vi "Main.vi"(11 "Module Admin":refnum<class "Delacor_lib_QMH_Module Admin.lvclass">) -> ()   [LabVIEW 2019, in "SME_Data_Acquisition.lvlib"]
doc: "This template is based off of the Queued Message Handler design pattern and the Queued Message Handler project template that ships with LabVIEW.\n\nThe main difference is that the queue is private to this module and communication between modules is performed via Broadcast and Request events.\n\nRequest events are wrapped in public API methods and are handled in the Event Handling Loop (EHL) of this VI. Any module can register for Broadcast events sent by this module. The EHL generates messages based on user interface actions.\n\nThe Message Handling Loop (MHL) processes messages generated by the EHL, or by other messages. The messages are string values, so new messages can be added easily to the Message Cases case structure in the MHL. Each message cluster can also provide an optional value for Message Data, which is a variant that can be converted to whatever message-specific data is required.\n_____\nBased on DQMH Project Template 7.0.1.1316."
uses:
  SME_Data_Acquisition.lvlib
  <vilib>/Delacor/Delacor QMH/Libraries/Module Admin_class/Delacor_lib_QMH_Module Admin.lvclass
  Module Data--cluster.ctl
  <vilib>/Delacor/Delacor QMH/Libraries/Message Queue_class/Delacor_lib_QMH_Message Queue.lvclass/Delacor_lib_QMH_Message Queue.ctl
  Stop Argument--cluster.ctl
  <vilib>/Delacor/Delacor QMH/Libraries/Module Admin_class/Delacor_lib_QMH_Module Admin.lvclass/Delacor_lib_QMH_Module Admin.ctl
  LogData Argument--cluster.ctl
  04 Class/Protocol/Protocol.lvclass
  <vilib>/Utility/sysdir.llb/System Directory Type.ctl
  <vilib>/Delacor/Delacor QMH/Libraries/Message Queue_class/Delacor_lib_QMH_Enqueue Message (Single).vi
  <vilib>/Delacor/Delacor QMH/Libraries/Module Admin_class/Delacor_lib_QMH_Get External Launch.vi
  <vilib>/Utility/file.llb/Write Delimited Spreadsheet (string).vi
  <vilib>/Delacor/Delacor QMH/Libraries/Message Queue_class/Delacor_lib_QMH_Message Queue.lvclass
panel:
  in  "Close":bool
  in  "LogEnable":bool caption="Data Log"
  in  "Com_Set":T1
  out "StatusLED":bool
  in  "Connect":bool
  in  "Protocol":enum16{"RS-232", "TCP/IP", "Modbus TCP/IP"}(ring)
  in  "Path":path caption="File Path"
  out "Data_Cluster":T2 {"Coil Temperature" format="%.2f"; "Channel 2 (c2)" format="%.3f"; "Channel 1 (c1)" format="%.3f"; "Freqency +45 Deg" format="%.7f"; "Freqency -45 Deg" format="%.7f"; "Freqency 0 Deg" format="%.7f"; "df frequency quotient" format="%.7f"; "Density" format="%.3f"; "Viscosity" format="%.3f"; "Damping Frequency" format="%.2g"; "Resonant Frequency" format="%.2f"; "Temperature" format="%.2f"}
  out "Table":string[][](table)
  out "Chart1":cluster{"Viscosity":dbl, "Temperature":dbl}(graph)
  out "Chart2":cluster{"Viscosity":dbl, "Temperature":dbl}(graph)
  out "Chart3":cluster{"Viscosity":dbl, "Temperature":dbl}(graph)
  out "ReceivedData":string
  out "error out":errorcluster
  out "Status":string
  in  "Simulate MHL Error":bool
  in  "Simulate EHL Error":bool
  # "Data Acquisition Interface"
  # "Other processes communicate with this Module via its Public API (wrappers for its Request Events).\n\nThis Module communicates with other processes via its Broadcast Events.\nAny process that wants to receive these messages can register for this module's Broadcast events."
  # "This template is for the DQMH framework. See the block diagram for more information on how to use this template."
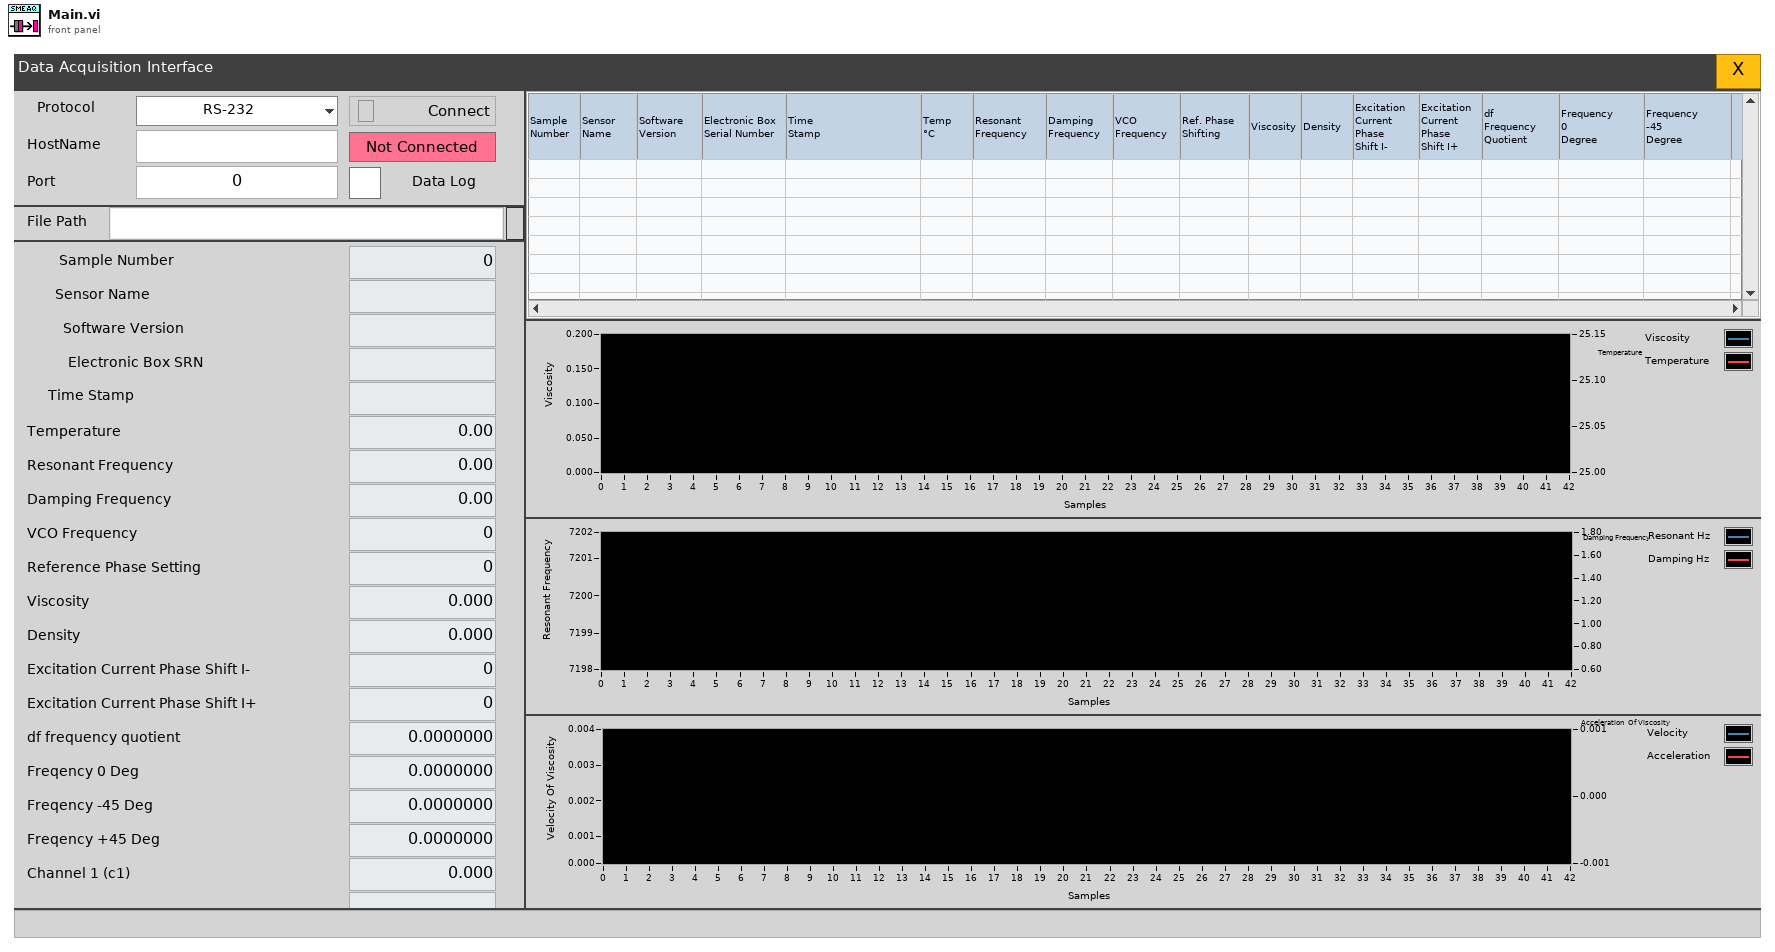
[diagram p1: front panel]
types:
  T1 = cluster{"HostName":string, "Port":dbl, "ComPort":string}
  T2 = cluster{"Sample Number":u16, "Sensor Name":string, "Software Version":string, "Electronic Box SRN":string, "Time Stamp":string, "Temperature":dbl, "Resonant Frequency":dbl, "Damping Frequency":dbl, "VCO Frequency":u16, "Reference Phase Setting":u16, "Viscosity":dbl, "Density":dbl, "Excitation Current Phase Shift I-":u16, "Excitation Current Phase Shift I+":u16, "df frequency quotient":dbl, "Freqency 0 Deg":dbl, "Freqency -45 Deg":dbl, "Freqency +45 Deg":dbl, "Channel 1 (c1)":dbl, "Channel 2 (c2)":dbl, "Coil Temperature":dbl, "Error State":u8}
  T3 = typedef "SME_Data_Acquisition.lvlib/Request Events--cluster.ctl" = cluster{"Stop Module":refnum<user-event>, "Show Panel":refnum<user-event>, "Hide Panel":refnum<user-event>, "Get Module Execution Status":refnum<user-event>, "Show Diagram":refnum<user-event>, "Private":cluster{"LogData":refnum<user-event>}}
  T4 = typedef "SME_Data_Acquisition.lvlib/Module Data--cluster.ctl" = cluster{"Status":string, "Path":refnum<vi>}
  T5 = cluster{"HostName":string, "Port":u16, "ComPort":string}
  T6 = enum32{"invalid lock state", "Not Locked", "Locked (No Password)", "Password-protected"}
  T7 = typedef "SME_Data_Acquisition.lvlib/Stop Argument--cluster.ctl" = cluster{"Origin":string, "Exit via Stop Module Req?":bool, "Wait for Module to stop?":bool}
  T8 = typedef "SME_Data_Acquisition.lvlib/LogData Argument--cluster.ctl" = cluster{"Data_Cluster":cluster{"Sample Number":u16, "Sensor Name":string, "Software Version":string, "Electronic Box SRN":string, "Time Stamp":string, "Temperature":dbl, "Resonant Frequency":dbl, "Damping Frequency":dbl, "VCO Frequency":u16, "Reference Phase Setting":u16, "Viscosity":dbl, "Density":dbl, "Excitation Current Phase Shift I-":u16, "Excitation Current Phase Shift I+":u16, "df frequency quotient":dbl, "Freqency 0 Deg":dbl, "Freqency -45 Deg":dbl, "Freqency +45 Deg":dbl, "Channel 1 (c1)":dbl, "Channel 2 (c2)":dbl, "Coil Temperature":dbl, "Error State":u8}}
  T9 = enum8{"Enabled", "Disabled", "Disabled and Grayed Out"}
  T10 = enum16{"Always On", "Always Off", "Off While Running"}
  T11 = enum32{"Invalid", "Standard", "Closed", "Hidden", "Minimized", "Maximized"}
  T12 = typedef "LVRectTypeDef.ctl" = cluster{"Left":i16, "Top":i16, "Right":i16, "Bottom":i16}
  T13 = typedef "System Directory Type.ctl" = i32
  T14 = cluster{"This VI":refnum<vi>, "ProtocolCls":refnum<class "Protocol.lvclass">, "Stream":string, "Table":refnum<vi>, "Data":string[][], "StatusLED":refnum<vi>, "LimitRowCount":u16, "Chart1":refnum<vi>, "Chart2":refnum<vi>, "Chart3":refnum<vi>, "Protocol":refnum<vi>, "Connect":refnum<vi>, "Com_Set":refnum<vi>, "Data_Cluster":refnum<vi>, "ConOpen":bool, "LogEnable":refnum<vi>}
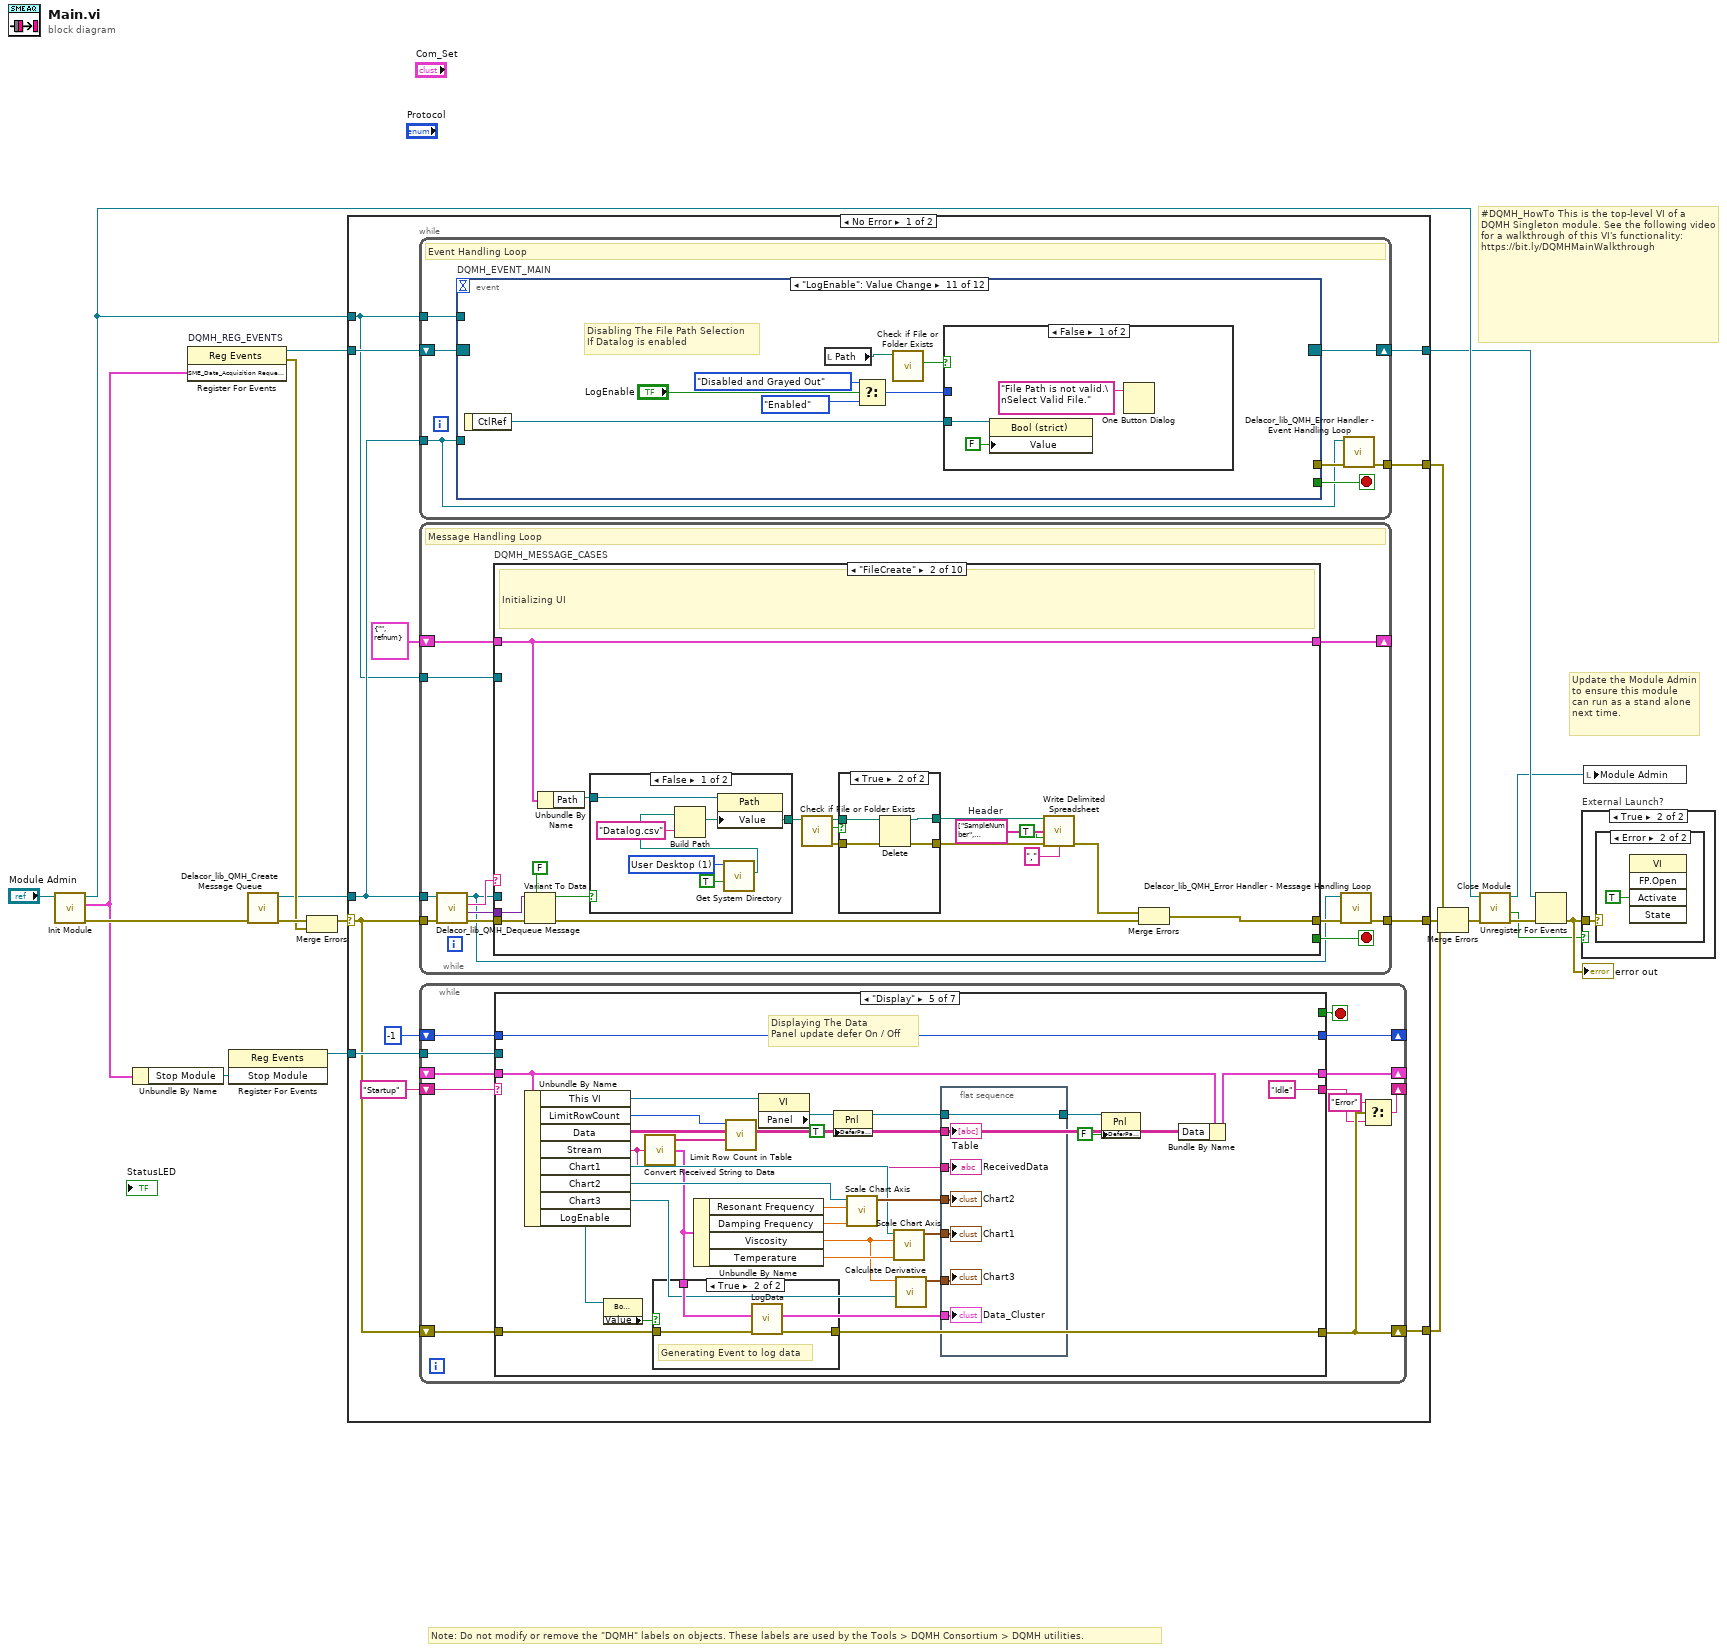
[diagram p0: block diagram]
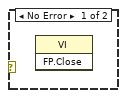
[diagram p3: hidden frame]
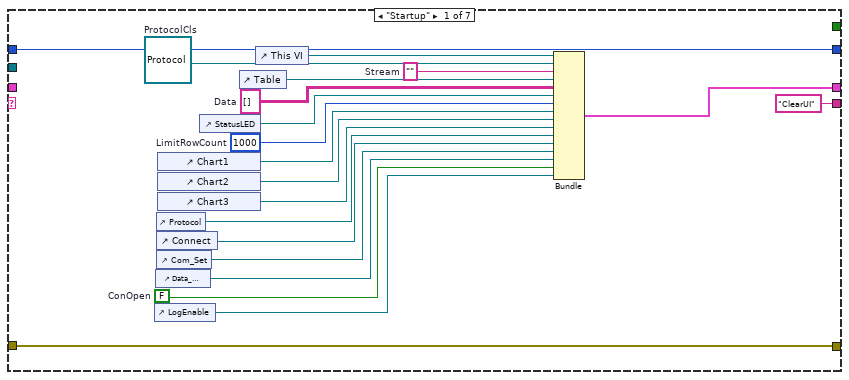
[diagram p4: hidden frame]
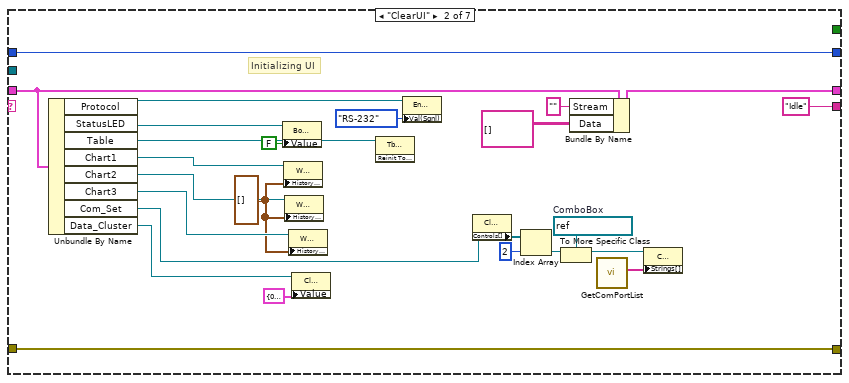
[diagram p5: hidden frame]
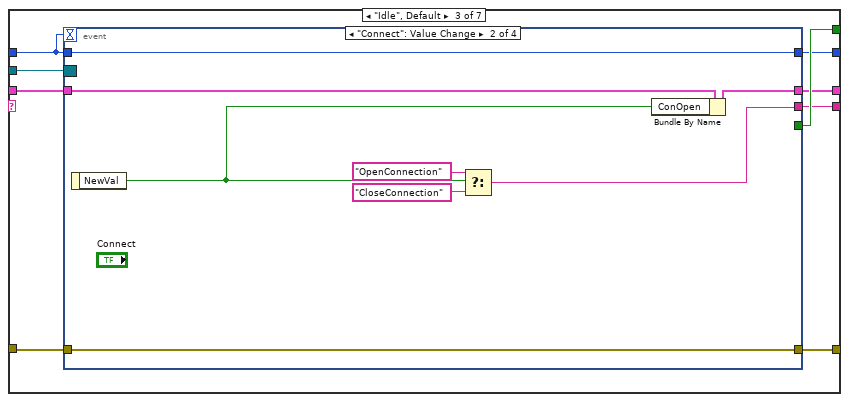
[diagram p6: hidden frame]
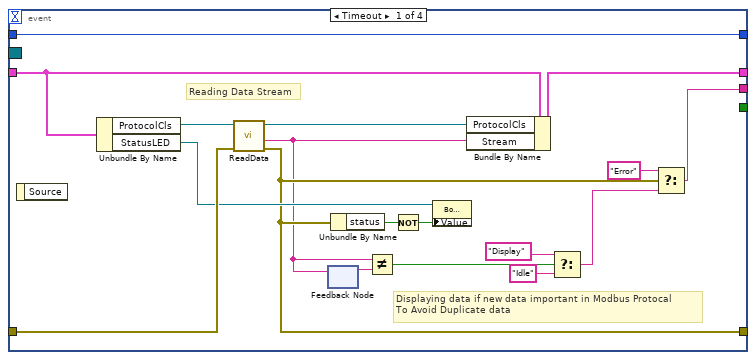
[diagram p7: hidden frame]
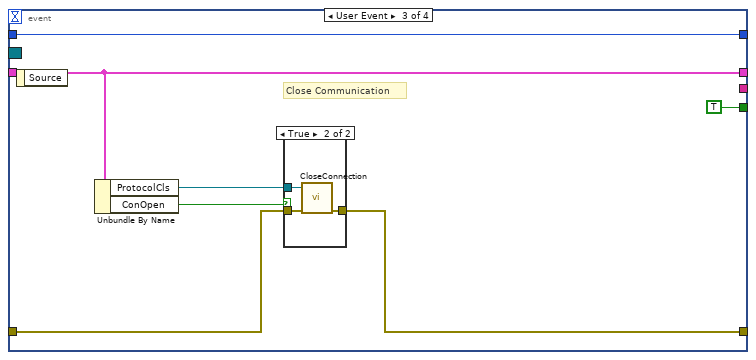
[diagram p8: hidden frame]
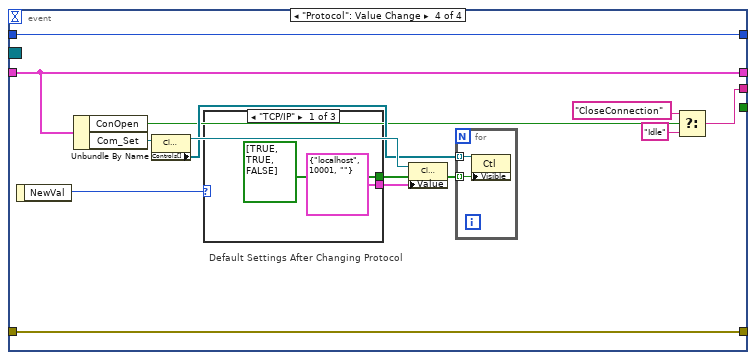
[diagram p10: hidden frame]
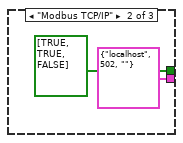
[diagram p11: hidden frame]
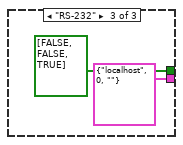
[diagram p12: hidden frame]
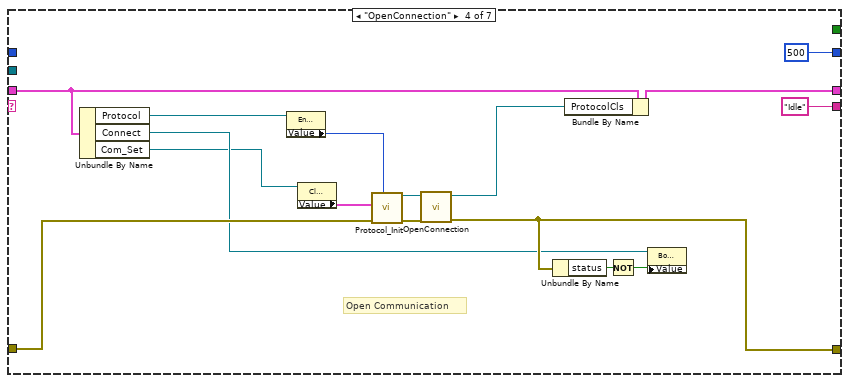
[diagram p13: hidden frame]
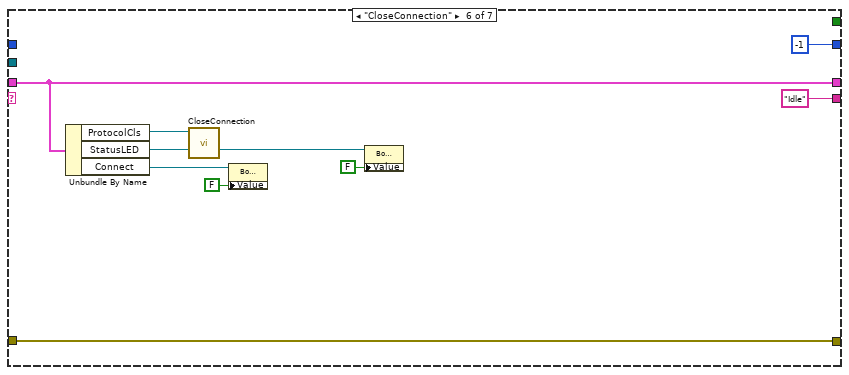
[diagram p15: hidden frame]
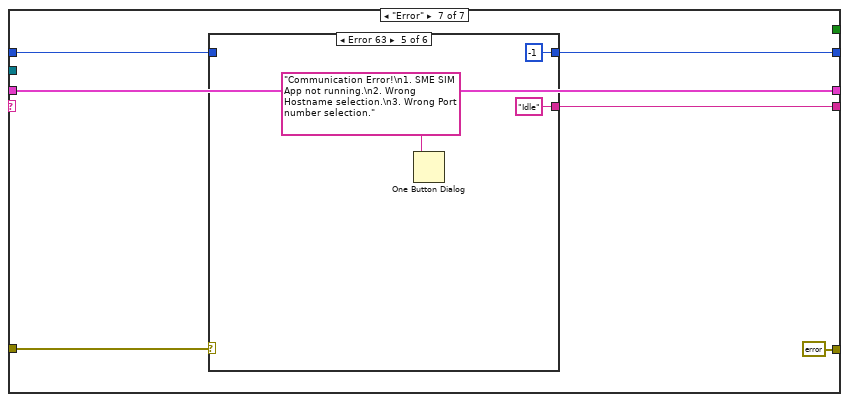
[diagram p16: hidden frame]
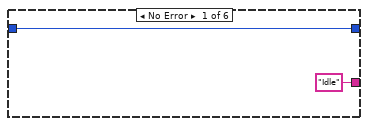
[diagram p17: hidden frame]
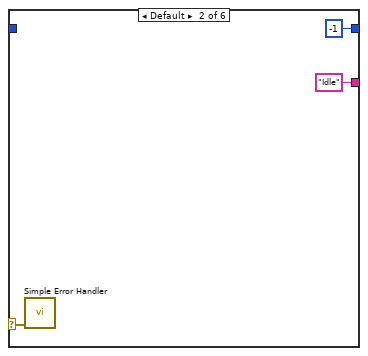
[diagram p18: hidden frame]
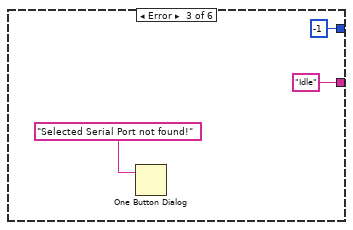
[diagram p19: hidden frame]
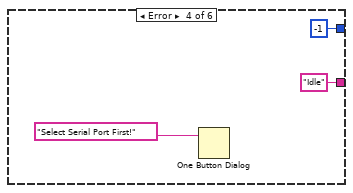
[diagram p20: hidden frame]
diagram:
  # "#DQMH_HowTo This is the top-level VI of a DQMH Singleton module. See the following video for a walkthrough of this VI's functionality: https://bit.ly/DQMHMainWalkthrough"
  # "Note: Do not modify or remove the \"DQMH\" labels on objects. These labels are used by the Tools > DQMH Consortium > DQMH utilities."
  # "Update the Module Admin to ensure this module can run as a stand alone next time."
  n1 = call "Init Module.vi"("Singleton Module Admin in"="Module Admin") -> ("error out"=w19:errorcluster, "SME_Data_Acquisition Request Events"=w4:T3, "Singleton Module Admin out"=w11:refnum<class "Delacor_lib_QMH_Module Admin.lvclass">)  [unwired: 8 in]
  n2 = Unbundle By Name(w4) -> ("Stop Module"=w3:refnum<user-event>)
  n3 = register-events "DQMH_REG_EVENTS"(w4) -> (reference out=w9:refnum<event-registration>, error out=w12:errorcluster)  [unwired: 2 in]
  n4 = register-events(w3) -> (reference out=w2:refnum<event-registration>)  [unwired: 2 in, 1 out]
  n5 = call <vilib>:"Delacor_lib_QMH_Create Message Queue.vi"("error in"=w19) -> ("error out"=w14:errorcluster, "Message Queue"=w8:refnum<class "Delacor_lib_QMH_Message Queue.lvclass">)  [unwired: 9 in]
  n6 = Merge Errors(w14, w12) -> (w13:errorcluster)
  n7 = case shown="No Error" w13 {
    selector: w13 -> [w22 w515]
    tunnel: [w32 w514] -> w20
    tunnel: [w30 w513] -> w10
    tunnel: w9 -> [w28 w513]
    tunnel: w8 -> [w27 w508]
    tunnel: [w31 _] -> w17
    tunnel: w11 -> [w26 w509]
    tunnel: w2 -> [w24 _]
    tunnel: [w21 _] -> w1
    frame No Error {
      n8 = while {
        tunnel: w27 -> [w245]
        shift-right: [w248] -> w30
        shift-left: w28 -> [w249]
        tunnel: [w250] -> w31
        tunnel: w26 -> [w246]
        stop <- w247 stop-if-true
        # "Event Handling Loop"
        n9 = event "DQMH_EVENT_MAIN" shown="[10] \"LogEnable\": Value Change" {
          selector: w249 -> [_ _ _ _ _ _ _ _ _ _ _ _]
          dyn-events: [_ _ _ _ _ _ _ _ _ _ _ _] -> w248
          timeout: _ -> [_ _ _ _ _ _ _ _ _ _ _ _]
          tunnel: [_ _ _ _ _ _ TRUE ("Discard?") _ _ _ _ _] -> w247
          tunnel: w245 -> [_ w259 _ _ _ _ w283 w290 w302 w316 _ w329]
          tunnel: [w257 w260 _ _ w266 _ w286 w292 w303 w311 _ _] -> w251
          tunnel: w246 -> [_ _ _ _ _ _ _ w289 w301 _ _ _]
          event "Simulate EHL Error": Value Change {
            # "#DQMH_HowTo The 'Simulate EHL Error' button  illustrates how the EHL handles errors. This event is instructional in nature and can be removed."
            # "This case simulates an error being generated by the EHL"
            n10 = event-data() -> ()  [unwired: 1 in, 1 out]
            n11 = call "Module Name--constant.vi"() -> ("Module Name"=w254:string)  [unwired: 11 in]
            n12 = Format Into String(format string="Simulated error originating at Event Handling Loop in %s", w254) -> (resulting string=w255:string)  [unwired: 2 in, 1 out]
            n13 = call <vilib>:"Error Cluster From Error Code.vi"("show call chain? (False)"=TRUE, "error message (\"\")"=w255, "error code (0)"=5000) -> ("error out"=w257:errorcluster)  [unwired: 6 in]
          }
          event "Simulate MHL Error": Value Change {
            # "#DQMH_HowTo The 'Simulate MHL Error' button  illustrates how the MHL handles errors. This event is instructional in nature and can be removed."
            # "This case simulates an error being generated by the MHL"
            n14 = event-data() -> ()  [unwired: 1 in, 1 out]
            n15 = call-poly <vilib>:"Delacor_lib_QMH_Enqueue Message (poly).vi"("Message"="Simulate MHL Error", "Message Queue in"=w259) -> ("error out"=w260:errorcluster)  [unwired: 8 in, 1 out]
          }
          event User Event {
            # "Show the panel of this VI, and send a status updated message to let listeners know."
            # "Another Module called the \"Show Panel\" API Method."
            n16 = event-data() -> ()  [unwired: 1 in, 1 out]
            n17 = control-ref of="This VI"() -> (w262:refnum<vi>)
            n18 = call "Open VI Panel.vi"("VI"=w262) -> ()  [unwired: 10 in, 1 out]
            n19 = call "Status Updated.vi"("Status"="Panel shown." ("format string")) -> ()  [unwired: 10 in, 1 out]
          }
          event User Event {
            # "Hide the panel of this VI, and send a status updated message to let listeners know."
            # "Another Module called the \"Hide Panel\" API Method."
            n20 = event-data() -> ()  [unwired: 1 in, 1 out]
            n21 = control-ref of="This VI"() -> (w264:refnum<vi>)
            n22 = call "Hide VI Panel.vi"("VI"=w264) -> ()  [unwired: 10 in, 1 out]
            n23 = call "Status Updated.vi"("Status"="Panel hidden." ("format string")) -> ()  [unwired: 10 in, 1 out]
          }
          event User Event {
            # "Another Module called the \"Get Module Execution Status\" API Method."
            n24 = event-data() -> ()  [unwired: 1 in, 1 out]
            n25 = call "Update Module Execution Status.vi"("Running?"=TRUE) -> ("error out"=w266:errorcluster)  [unwired: 10 in]
          }
          event User Event {
            # "Another Module called the \"Show Diagram\" API Method. This event is used for debugging."
            n26 = event-data() -> ()  [unwired: 1 in, 1 out]
            n27 = disable-structure shown="RUN_TIME_ENGINE==False" {
              frame condition #0 (active) {
                # "functionality not available in exe"
                n28 = invoke on="Invoke Node" class="VI" method="Lock State.Get"() -> (error out=w272:errorcluster, "Get Lock State"=w271:T6, "pwd in cache"=w268:bool)  [unwired: 4 in, 1 out]
                n29 = Equal?(x=T6."Password-protected", y=w271) -> (x = y?=w269:bool)
                n30 = Compound Arithmetic op=AND(w269, invert w268) -> (w267:bool)
                n31 = case shown="False" w267 {
                  tunnel: w272 -> [w275 _]
                  frame False {
                    n32 = property on="Property Node" class="VI"(error in=w275, "BDWin.Open"=TRUE ("Block Diagram Window:Open")) -> ()  [unwired: 1 in, 2 out]
                    n33 = call "Status Updated.vi"("Status"="Block Diagram shown." ("format string")) -> ()  [unwired: 10 in, 1 out]
                  }
                  frame True {
                    # "Password-protected VI, and the password is not in the cache. Do not show the diagram."
                  }
                }
              }
              frame condition #1 {
              }
            }
          }
          event User Event {
            # "The Stop Module Event can get fired from the Exit message in the MHL. The queue gets destroyed in that case. If the queue no longer exists, the Enqueue Exit as a priority message will return error 1. It is safe to ignore, because the module is already exiting."
            # "Another Module called the \"Stop Module\" API Method  or the Message Handling Loop below."
            n34 = event-data() -> ("Origin"=w282:string, "Exit via Stop Module Req?"=w278:bool, "Wait for Module to stop?"=w277:bool)  [unwired: 1 in]
            n35 = local write "Status"(w282) -> ()
            n36 = Bundle By Name(cluster=T7 {"Origin"="", "Exit via Stop Module Req?"=FALSE, "Wait for Module to stop?"=FALSE} ("Stop Argument"), "Exit via Stop Module Req?"=w278, "Wait for Module to stop?"=w277) -> (w276:T7)
            n37 = call-poly <vilib>:"Delacor_lib_QMH_Enqueue Message (poly).vi"("Priority Message? (F)"=TRUE, "Message Data"=w276, "Message"="Exit", "Message Queue in"=w283) -> ("error out"=w287:errorcluster)  [unwired: 6 in, 1 out]
            n38 = call <vilib>:"Clear Errors.vi"("error in (no error)"=w287, "specific error code to clear (0: all)"=1) -> ("error out"=w286:errorcluster)  [unwired: 4 in, 1 out]
          }
          event Panel Close? {
            w291 = TRUE  # Discard the event, the MHL is responsible for closing and stopping this VI.
            # "Hide the panel or send the 'Exit' message if the user clicks the 'X' on the module main VI panel."
            n39 = event-data() -> ()  [unwired: 1 in, 1 out]
            n40 = property on="Property Node" class="Module Admin"(reference=w289) -> ("Accessors:External Launch"=w288:bool)  [unwired: 1 in, 2 out]
            n41 = case shown="False" w288 {
              tunnel: w290 -> [_ w298]
              tunnel: [_ w299] -> w292
              frame True {
                # "If externally launched, clicking the 'X' hides the panel, but doesn't close it."
                n42 = control-ref of="This VI"() -> (w295:refnum<vi>)
                n43 = call "Hide VI Panel.vi"("VI"=w295) -> ("error out"=w293:errorcluster)  [unwired: 10 in]
                n44 = call "Status Updated.vi"("error in"=w293, "Status"="Panel hidden." ("format string")) -> ()  [unwired: 9 in, 1 out]
              }
              frame False {
                # "If run as a stand-alone VI, clicking the panel 'X' stops the VI."
                n45 = call-poly <vilib>:"Delacor_lib_QMH_Enqueue Message (poly).vi"("Priority Message? (F)"=TRUE, "Message"="Exit", "Message Queue in"=w298) -> ("error out"=w299:errorcluster)  [unwired: 7 in, 1 out]
              }
            }
            n46 = event-data ("Event Filter Node")("Discard?"=w291) -> ()  [unwired: 1 in, 1 out]
          }
          event "Close": Value Change {
            # "Hide the panel or send the 'Exit' message if the user clicks the 'X' on the module main VI panel."
            n47 = event-data() -> ()  [unwired: 1 in, 1 out]
            n48 = property on="Property Node" class="Module Admin"(reference=w301) -> ("Accessors:External Launch"=w300:bool)  [unwired: 1 in, 2 out]
            n49 = case shown="False" w300 {
              tunnel: w302 -> [_ w309]
              tunnel: [_ w310] -> w303
              frame True {
                # "If externally launched, clicking the 'X' hides the panel, but doesn't close it."
                n50 = control-ref of="This VI"() -> (w306:refnum<vi>)
                n51 = call "Hide VI Panel.vi"("VI"=w306) -> ("error out"=w304:errorcluster)  [unwired: 10 in]
                n52 = call "Status Updated.vi"("error in"=w304, "Status"="Panel hidden." ("format string")) -> ()  [unwired: 9 in, 1 out]
              }
              frame False {
                # "If run as a stand-alone VI, clicking the panel 'X' stops the VI."
                n53 = call-poly <vilib>:"Delacor_lib_QMH_Enqueue Message (poly).vi"("Priority Message? (F)"=TRUE, "Message"="Exit", "Message Queue in"=w309) -> ("error out"=w310:errorcluster)  [unwired: 7 in, 1 out]
              }
            }
          }
          event User Event {
            # "This module called the \"Private.LogData\" private request."
            n54 = event-data() -> ("Data_Cluster"=w312:T2)  [unwired: 1 in]
            n55 = Bundle(cluster=T8 {"Data_Cluster"={"Sample Number"=0, "Sensor Name"="", "Software Version"="", "Electronic Box SRN"="", "Time Stamp"="", "Temperature"=0.0, "Resonant Frequency"=0.0, "Damping Frequency"=0.0, "VCO Frequency"=0, "Reference Phase Setting"=0, "Viscosity"=0.0, "Density"=0.0, "Excitation Current Phase Shift I-"=0, "Excitation Current Phase Shift I+"=0, "df frequency quotient"=0.0, "Freqency 0 Deg"=0.0, "Freqency -45 Deg"=0.0, "Freqency +45 Deg"=0.0, "Channel 1 (c1)"=0.0, "Channel 2 (c2)"=0.0, "Coil Temperature"=0.0, "Error State"=0}} ("LogData Argument"), "Data_Cluster"=w312) -> (w313:T8)
            n56 = call-poly <vilib>:"Delacor_lib_QMH_Enqueue Message (poly).vi"("Message Data"=w313, "Message"="LogData", "Message Queue in"=w316) -> ("error out"=w311:errorcluster)  [unwired: 7 in, 1 out]
          }
          event "LogEnable": Value Change {
            # "Disabling The File Path Selection\nIf Datalog is enabled"
            n57 = event-data() -> ("CtlRef"=w317:refnum<vi>)  [unwired: 1 in]
            n58 = local read "Path"() -> (w319:path)
            n59 = Select(t=T9."Disabled and Grayed Out" ("Disabled"), s="LogEnable", f=T9."Enabled" ("Disabled")) -> (s? t:f=w320:T9)
            n60 = call <vilib>:"Check if File or Folder Exists.vi"("path"=w319) -> ("file or folder exists?"=w318:bool)  [unwired: 8 in, 2 out]
            n61 = case shown="False" w318 {
              tunnel: w320 -> [_ w327]
              tunnel: w317 -> [w325 _]
              frame False {
                n62 = property class="Bool (strict)"(reference=w325, "Value"=FALSE) -> ()  [unwired: 1 in, 2 out]
                n63 = One Button Dialog(message="File Path is not valid.\nSelect Valid File.") -> ()  [unwired: 1 in, 1 out]
              }
              frame True {
                n64 = property on="Path" class="Path"("DisabledEnum"=w327) -> ()  [unwired: 2 in, 2 out]
              }
            }
          }
          event "Path": Value Change {
            w328 = TRUE  # PathChangedByUser
            # "Sending"
            n65 = event-data() -> ()  [unwired: 1 in, 1 out]
            n66 = call-poly <vilib>:"Delacor_lib_QMH_Enqueue Message (poly).vi"("Message Data"=w328, "Message"="FileCreate", "Message Queue in"=w329) -> ()  [unwired: 7 in, 2 out]
          }
        }
        n67 = call-dynamic "Delacor_lib_QMH_Error Handler - Event Handling Loop.vi"("error in"=w251, "Message Queue in"=w245) -> ("dup error in"=w250:errorcluster)  [unwired: 8 in, 1 out]
      }
      n68 = while {
        tunnel: w27 -> [w331]
        shift-right: [w339] -> _
        shift-left: T4 {"Status"="", "Path"=refnum} ("Data Cluster") -> [w340]
        tunnel: w22 -> [w342]
        tunnel: [w334] -> w32
        tunnel: w26 -> [w335]
        stop <- w338 stop-if-true
        # "Message Handling Loop"
        n69 = call-dynamic "Delacor_lib_QMH_Dequeue Message.vi"("error in"=w342, "Message Queue in"=w331) -> ("error out"=w341:errorcluster, "Message Data"=w336:variant, "Message"=w337:string, "Message Queue out"=w332:refnum<class "Delacor_lib_QMH_Message Queue.lvclass">)  [unwired: 6 in]
        n70 = case "DQMH_MESSAGE_CASES" shown="\"FileCreate\"" w337 {
          selector: w337 -> [_ _ _ _ _ _ _ _ _ w503]
          tunnel: w332 -> [w359 _ _ _ _ _ _ w469 w491 _]
          tunnel: w341 -> [w375 w384 w410 w451 w454 w456 w465 w476 w497 w506]
          tunnel: [w358 w379 w410 w412 w453 w456 w464 w472 w492 w507] -> w333
          tunnel: w340 -> [w367 w394 w409 w446 w452 w455 w462 w471 w490 w504]
          tunnel: [w366 w394 w409 w446 w452 w455 w462 w471 w490 w504] -> w339
          tunnel: [_ _ _ _ _ _ _ _ w489 _] -> w338
          tunnel: w336 -> [_ w382 _ w449 _ _ _ w470 w488 _]
          tunnel: w335 -> [w368 _ _ _ _ _ _ w468 w483 _]
          frame "Initialize" {
            w362 = "Initial Message" ("Initial Message")
            # "Enable Scrollbar on the pane if pane size is lower than data cluster size"
            # "Initialize - Any operation that needs to be done before the module can receive messages. Synchronize Caller Events.vi will inform Start Module.vi that the module has launched and is ready to receive messages. Module Did Init.vi will broadcast that the module initialized."
            n71 = call "Synchronize Caller Events.vi"("error in"=w375, "Singleton Module Admin in"=w368) -> ("error out"=w374:errorcluster, "Singleton Module Admin out"=w363:refnum<class "Delacor_lib_QMH_Module Admin.lvclass">)  [unwired: 8 in]
            n72 = control-ref of="Pane 4"() -> (w347:refnum<vi>)
            n73 = property on="Property Node" class="Module Admin"(reference=w363) -> ("Accessors:External Launch"=w357:bool)  [unwired: 1 in, 2 out]
            n74 = property on="Property Node" class="Pane"(reference=w347) -> (reference out=w350:refnum<vi>, "ContentBnds"=w353:T12)  [unwired: 1 in, 1 out]
            n75 = property on="Data_Cluster" class="Clust (strict)"() -> ("Bounds Rect"=w354:T12)  [unwired: 2 in, 2 out]
            n76 = Unbundle By Name(w354) -> ("Bottom"=w352:i16)
            n77 = Select(t=T11."Hidden" ("State"), s=w357, f=T11."Maximized" ("State")) -> (s? t:f=w369:T11)
            n78 = Unbundle By Name(w353) -> ("Bottom"=w351:i16)
            n79 = Not(x=w357) -> (.not. x?=w356:bool)
            n80 = call "Module Name--constant.vi"() -> ("Module Name"=w373:string)  [unwired: 11 in]
            n81 = Less?(x=w351, y=w352) -> (x < y?=w349:bool)
            n82 = property on="Close" class="Bool"("Visible"=w356) -> ()  [unwired: 2 in, 2 out]
            n83 = property on="Property Node" class="VI"("Front Panel.Title"=w373) -> (reference out=w372:refnum<vi>, error out=w376:errorcluster)  [unwired: 2 in]
            n84 = call "Module Name--constant.vi"() -> ("Module Name"=w364:string)  [unwired: 11 in]
            n85 = invoke on="Invoke Node" class="VI" method="FP.Open"(reference=w372, error in=w376, "State"=w369) -> ()  [unwired: 2 in, 5 out]
            n86 = call "Module Did Init.vi"("error in"=w374, "Initialized?"=TRUE, "Origin"=w364) -> ("error out"=w360:errorcluster)  [unwired: 8 in]
            n87 = Select(t=T10."Always On" ("Vertical Scrollbar Visibility"), s=w349, f=T10."Always Off" ("Vertical Scrollbar Visibility")) -> (s? t:f=w348:T10)
            n88 = property on="Property Node" class="Pane"(reference=w350, "VertScrollbarVisibility"=w348) -> ()  [unwired: 1 in, 2 out]
            n89 = control-ref of="Path"() -> (w344:refnum<vi>)
            n90 = call-poly <vilib>:"Delacor_lib_QMH_Enqueue Message (poly).vi"("error in"=w360, "Message Data"=FALSE, "Message"="FileCreate", "Message Queue in"=w359) -> ("error out"=w358:errorcluster)  [unwired: 6 in, 1 out]
            n91 = property class="Path"(reference=w344, "DisabledEnum"=T9."Enabled" ("Disabled")) -> ()  [unwired: 1 in, 2 out]
            n92 = Bundle By Name(cluster=w367, "Status"=w362, "Path"=w344) -> (w366:T4)
            "Status" <- w362
          }
          frame "FileCreate" {
            w388 = string[] ["SampleNumber", "SensorName", "SoftwareVersion", "ElectronicBoxSR", "TimeStamp", "Temperature", "ResonantFrequency", "DampingFrequency", "VCOFrequency", "RefPhaseShifting", "Viscosity", "Density", "ExcitationCurrentPhaseShift I-", "ExcitationCurrentPhaseShift I+", "dfFrequencyQuotient", "Frequency0Degree", "Frequency-45Degree", "Frequency+45Degree", "Channel1c1", "Channel2c2", "CoilTemperature", "ErrorCode"]  # Header
            # "Initializing UI"
            n93 = Variant To Data(error in=w384, type=FALSE, Variant=w382) -> (data=w380:bool, error out=w383:errorcluster)
            n94 = Unbundle By Name(w394) -> ("Path"=w391:refnum<vi>)
            n95 = case shown="False" w380 {
              tunnel: w391 -> [w399 w402]
              tunnel: [w398 w401] -> w390
              frame False {
                w397 = T13 1 items=["User Home"=0, "User Desktop"=1, "User Documents"=2, "User Application Data"=3, "User Preferences"=4, "User Temporary"=5, "Public Documents"=6, "Public Application Data"=7, "Public Preferences"=8, "Public Cache"=13, "System Core Libraries"=9, "System Installed Libraries"=10, "Application Files"=11, "Boot Volume Root"=12] ("system directory type")
                n96 = call <vilib>:"Get System Directory.vi"("create directory if not found? (F)"=TRUE, "system directory type"=w397) -> ("system directory"=w395:path)  [unwired: 9 in]
                n97 = Build Path(base path=w395, name or relative path="Datalog.csv") -> (appended path=w398:path)
                n98 = property class="Path"(reference=w399, "Value"=w398) -> ()  [unwired: 1 in, 2 out]
              }
              frame True {
                n99 = property class="Path"(reference=w402) -> ("Value"=w401:path)  [unwired: 1 in, 2 out]
              }
            }
            n100 = call <vilib>:"Check if File or Folder Exists.vi"("path"=w390) -> ("error out"=w377:errorcluster, "file or folder exists?"=w393:bool, "dup path"=w392:path)  [unwired: 8 in]
            n101 = case shown="True" w393 {
              tunnel: w392 -> [w404 w408]
              tunnel: [w404 w407] -> w389
              tunnel: [w403 w406] -> w386
              tunnel: w377 -> [w403 w405]
              frame False {
              }
              frame True {
                n102 = Delete(path (use dialog)=w408, error in=w405) -> (deleted path=w407:path, error out=w406:errorcluster)  [unwired: 3 in, 1 out]
              }
            }
            n103 = call-poly <vilib>:"Write Delimited Spreadsheet.vi"("file path (dialog if empty)"=w389, "1D data"=w388, "append to file? (new file:F)"=TRUE, "error in (no error)"=w386, "delimiter (\\t)"="," ("delimiter (\\t)")) -> ("error out"=w378:errorcluster)  [unwired: 9 in, 1 out]
            n104 = Merge Errors(w378, w383) -> (w379:errorcluster)
          }
          frame "---Module Specific---" {
            # "Separator -- The following cases handle messages specific to this Module."
          }
          frame "LogData" {
            # "This even is generated by helper loop to log data."
            n105 = Variant To Data(error in=w451, type=T8 {"Data_Cluster"={"Sample Number"=0, "Sensor Name"="", "Software Version"="", "Electronic Box SRN"="", "Time Stamp"="", "Temperature"=0.0, "Resonant Frequency"=0.0, "Damping Frequency"=0.0, "VCO Frequency"=0, "Reference Phase Setting"=0, "Viscosity"=0.0, "Density"=0.0, "Excitation Current Phase Shift I-"=0, "Excitation Current Phase Shift I+"=0, "df frequency quotient"=0.0, "Freqency 0 Deg"=0.0, "Freqency -45 Deg"=0.0, "Freqency +45 Deg"=0.0, "Channel 1 (c1)"=0.0, "Channel 2 (c2)"=0.0, "Coil Temperature"=0.0, "Error State"=0}} ("LogData Argument"), Variant=w449) -> (data=w447:T8, error out=w450:errorcluster)
            n106 = Unbundle By Name(w447) -> ("Data_Cluster"=w420:T2)
            n107 = Unbundle By Name(w446) -> ("Path"=w419:refnum<vi>)
            n108 = property class="Path"(reference=w419) -> ("Value"=w418:path)  [unwired: 1 in, 2 out]
            n109 = Unbundle(w420) -> ("Sample Number"=w442:u16, "Sensor Name"=w424:string, "Software Version"=w423:string, "Electronic Box SRN"=w422:string, "Time Stamp"=w421:string, "Temperature"=w441:dbl, "Resonant Frequency"=w440:dbl, "Damping Frequency"=w439:dbl, "VCO Frequency"=w438:u16, "Reference Phase Setting"=w437:u16, "Viscosity"=w436:dbl, "Density"=w435:dbl, "Excitation Current Phase Shift I-"=w434:u16, "Excitation Current Phase Shift I+"=w433:u16, "df frequency quotient"=w432:dbl, "Freqency 0 Deg"=w431:dbl, "Freqency -45 Deg"=w430:dbl, "Freqency +45 Deg"=w429:dbl, "Channel 1 (c1)"=w428:dbl, "Channel 2 (c2)"=w427:dbl, "Coil Temperature"=w426:dbl, "Error State"=w425:u8)
            n110 = Format Into String(format string="%d,%S,%S,%S,%S,%0.2f,%0.2f,%0.2f,%d,%d,%0.3f,%0.3f,%d,%d,%0.7f,%0.7f,%0.7f,%0.7f,%0.3f,%0.3f,%0.3f,%d", w442, w424, w423, w422, w421, w441, w440, w439, w438, w437, w436, w435, w434, w433, w432, w431, w430, w429, w428, w427, w426, w425) -> (resulting string=w417:string)  [unwired: 2 in, 1 out]
            n111 = Spreadsheet String To Array(delimiter (Tab)=",", format string="", spreadsheet string=w417, array type (2D Dbl)=string[] [] ("appended array")) -> (array=w413:string[])
            n112 = call-poly <vilib>:"Write Delimited Spreadsheet.vi"("file path (dialog if empty)"=w418, "1D data"=w413, "append to file? (new file:F)"=TRUE, "delimiter (\\t)"="," ("delimiter (\\t)")) -> ("error out"=w411:errorcluster)  [unwired: 10 in, 1 out]
            n113 = Merge Errors(w411, w450) -> (w412:errorcluster)
          }
          frame "---Copy This Frame---" {
            # "Duplicate this frame when creating new messages.  Change this comment in the duplicated frame to describe this message."
            n114 = Merge Errors(w454) -> (w453:errorcluster)
          }
          frame "---Exit and Error Handling---" {
            # "Separator - The following cases handle errors and exit messages."
          }
          frame "Simulate MHL Error" {
            # "#DQMH_HowTo The 'Simulate MHL Error' button  illustrates how the MHL handles errors. This event is instructional in nature and can be removed."
            # "Simulate an error occurring at the MHL"
            n115 = call "Module Name--constant.vi"() -> ("Module Name"=w458:string)  [unwired: 11 in]
            n116 = Format Into String(format string="Simulated error originating at Message Handling Loop in %s", w458) -> (resulting string=w459:string)  [unwired: 2 in, 1 out]
            n117 = call <vilib>:"Error Cluster From Error Code.vi"("show call chain? (False)"=TRUE, "error message (\"\")"=w459, "error code (0)"=5001) -> ("error out"=w463:errorcluster)  [unwired: 6 in]
            n118 = Merge Errors(w465, w463) -> (w464:errorcluster)
          }
          frame "Error" {
            # "#CodeRecommended - If the module is running in standalone mode (External Launch = FALSE), this code will pop up an error dialog and call the 'Exit' message if an error occurs. Add more fine-grained error management here."
            # "Error - Check the error message data and respond accordingly. This message is sent by the \"Error Handler\" VIs at the end of each loop in this application."
            n119 = property on="Property Node" class="Module Admin"(reference=w468) -> ("Accessors:External Launch"=w467:bool)  [unwired: 1 in, 2 out]
            n120 = Variant To Data(error in=w476, type=errorcluster {"status"=FALSE, "code"=0, "source"=""} ("error constant"), Variant=w470) -> (data=w466:errorcluster, error out=w474:errorcluster)
            n121 = local write "error out"(w466) -> ()
            n122 = call "Error Reported.vi"("Error"=w466) -> ()  [unwired: 10 in, 1 out]
            n123 = case shown="False" w467 {
              tunnel: [w481 _] -> w473
              tunnel: w469 -> [w479 _]
              tunnel: w466 -> [w480 _]
              frame False {
                n124 = disable-structure shown="Default" {
                  disable-tunnel: w480 -> [w482 _]
                  frame condition #0 (active) {
                    # "If the module is running standalone, then pop up an error dialog and call the \"Exit\" message."
                    n125 = call <vilib>:"Simple Error Handler.vi"("error in (no error)"=w482) -> ()  [unwired: 4 in, 5 out]
                  }
                  frame condition #1 {
                    # "To prevent the Simple Error Handler VI from being loaded (e.g. when deploying to a Real-Time target), add the Conditional Disable Symbol \"DQMH_Disable_SEH\" to your project and set it to TRUE."
                  }
                }
                n126 = call-poly <vilib>:"Delacor_lib_QMH_Enqueue Message (poly).vi"("Priority Message? (F)"=TRUE, "Message"="Exit", "Message Queue in"=w479) -> ("error out"=w481:errorcluster)  [unwired: 7 in, 1 out]
              }
              frame True {
                # "If the module was launched externally, calling the Error Reported broadcast VI is the only action performed by the \"Error\" message. The module's caller can then process the error appropriately."
              }
            }
            n127 = Merge Errors(w474, w473) -> (w472:errorcluster)
          }
          frame "Exit" {
            w487 = 91  # 91: not all Exit messages will have an argument
            w489 = TRUE  # Stop the VI
            # "Release the message queue reference"
            # "#CodeNeeded - Add any required cleanup code here."
            # "Exit - Exit the application."
            n128 = Variant To Data(error in=w497, type=T7 {"Origin"="", "Exit via Stop Module Req?"=FALSE, "Wait for Module to stop?"=FALSE} ("Stop Argument"), Variant=w488) -> (data=w485:T7, error out=w494:errorcluster)
            n129 = call <vilib>:"Clear Errors.vi"("error in (no error)"=w494, "specific error code to clear (0: all)"=w487) -> ("error out"=w496:errorcluster)  [unwired: 4 in, 1 out]
            n130 = control-ref of="This VI"() -> (w484:refnum<vi>)
            n131 = call-dynamic "Delacor_lib_QMH_Release Message Queue.vi"("error in"=w496, "Message Queue"=w491) -> ("error out"=w495:errorcluster)  [unwired: 9 in]
            n132 = call "Handle Exit.vi"("Stop Argument"=w485, "Admin in"=w483, "VI reference"=w484) -> ("error out"=w493:errorcluster)  [unwired: 7 in, 1 out]
            n133 = Merge Errors(w495, w493) -> (w492:errorcluster)
            n134 = call "Error Reported.vi"("Error"=w492) -> ()  [unwired: 10 in, 1 out]
          }
          frame Default {
            # "'Default' case only runs if there is a message that isn't defined in any of the other cases.  Output a programming error."
            n135 = call "Module Name--constant.vi"() -> ("Module Name"=w502:string)  [unwired: 11 in]
            n136 = Format Into String(format string="The invalid message string \"%s\" was received in the Message Handling Loop for module \"%s\".", w503, w502) -> (resulting string=w498:string)  [unwired: 2 in, 1 out]
            n137 = call <vilib>:"Error Cluster From Error Code.vi"("show call chain? (False)"=TRUE, "error message (\"\")"=w498, "error code (0)"=1) -> ("error out"=w505:errorcluster)  [unwired: 6 in]
            n138 = Merge Errors(w506, w505) -> (w507:errorcluster)
          }
        }
        n139 = call-dynamic "Delacor_lib_QMH_Error Handler - Message Handling Loop.vi"("error in"=w333, "Message Queue in"=w332) -> ("dup error in"=w334:errorcluster)  [unwired: 8 in, 1 out]
      }
      n140 = while {
        shift-right: [w41] -> _
        shift-left: -1 -> [w42]
        tunnel: w24 -> [w44]
        shift-right: [w33] -> _
        shift-left: "Startup" -> [w40]
        shift-right: [w39] -> _
        shift-left: _ -> [w38]
        shift-right: [w36] -> w21
        shift-left: w22 -> [w37]
        stop <- w43 stop-if-true
        n141 = case shown="\"Display\"" w40 {
          tunnel: w44 -> [_ _ w98 _ _ _ _]
          tunnel: [_ _ w97 _ _ _ _] -> w43
          tunnel: w42 -> [w63 w88 w96 _ w202 _ w225]
          tunnel: [w63 w88 w95 500 w202 -1 w224] -> w41
          tunnel: ["ClearUI" "Idle" ("t") w94 "Idle" "Idle" "Idle" w223] -> w34
          tunnel: [w61 w83 w92 w166 w198 w220 w228] -> w39
          tunnel: w38 -> [_ w86 w93 w160 w201 w220 w228]
          tunnel: w37 -> [w57 w89 w91 w164 w186 w218 w226]
          tunnel: [w57 w89 w90 w163 w187 w218 errorcluster {"status"=FALSE, "code"=0, "source"=""} ("error IO")] -> w36
          frame "Startup" {
            w46 = FALSE  # ConOpen
            w55 = u16 1000  # LimitRowCount
            w58 = string[][] []  # Data
            w60 = ""  # Stream
            w62 = refnum<class "Protocol.lvclass"> refnum  # ProtocolCls
            n142 = control-ref of="LogEnable"() -> (w45:refnum<vi>)
            n143 = control-ref of="Data_Cluster"() -> (w47:refnum<vi>)
            n144 = control-ref of="Protocol"() -> (w50:refnum<vi>)
            n145 = control-ref of="Connect"() -> (w49:refnum<vi>)
            n146 = control-ref of="Com_Set"() -> (w48:refnum<vi>)
            n147 = control-ref of="Chart1"() -> (w53:refnum<vi>)
            n148 = control-ref of="Chart2"() -> (w52:refnum<vi>)
            n149 = control-ref of="Chart3"() -> (w51:refnum<vi>)
            n150 = control-ref of="StatusLED"() -> (w56:refnum<vi>)
            n151 = control-ref of="Table"() -> (w59:refnum<vi>)
            n152 = control-ref of="This VI"() -> (w54:refnum<vi>)
            n153 = Bundle("This VI"=w54, "ProtocolCls"=w62, "Stream"=w60, "Table"=w59, "Data"=w58, "StatusLED"=w56, "LimitRowCount"=w55, "Chart1"=w53, "Chart2"=w52, "Chart3"=w51, "Protocol"=w50, "Connect"=w49, "Com_Set"=w48, "Data_Cluster"=w47, "ConOpen"=w46, "LogEnable"=w45) -> (w61:T14)  [unwired: 1 in]
          }
          frame "ClearUI" {
            w73 = refnum<vi> refnum  # ComboBox
            w76 = cluster{"Viscosity":dbl, "Temperature":dbl}[] [] ("History Data")
            # "Initializing UI"
            n154 = Unbundle By Name(w86) -> ("Protocol"=w68:refnum<vi>, "StatusLED"=w85:refnum<vi>, "Table"=w81:refnum<vi>, "Chart1"=w79:refnum<vi>, "Chart2"=w78:refnum<vi>, "Chart3"=w77:refnum<vi>, "Com_Set"=w67:refnum<vi>, "Data_Cluster"=w66:refnum<vi>)
            n155 = property class="Bool (strict)"(reference=w85, "Value"=FALSE) -> ()  [unwired: 1 in, 2 out]
            n156 = property class="WFChart (strict)"(reference=w79, "History Data"=w76) -> ()  [unwired: 1 in, 2 out]
            n157 = property class="WFChart (strict)"(reference=w78, "History Data"=w76) -> ()  [unwired: 1 in, 2 out]
            n158 = property class="WFChart (strict)"(reference=w77, "History Data"=w76) -> ()  [unwired: 1 in, 2 out]
            n159 = property class="Clust (strict)"(reference=w66, "Value"=T2 {"Sample Number"=0, "Sensor Name"="", "Software Version"="", "Electronic Box SRN"="", "Time Stamp"="", "Temperature"=0.0, "Resonant Frequency"=0.0, "Damping Frequency"=0.0, "VCO Frequency"=0, "Reference Phase Setting"=0, "Viscosity"=0.0, "Density"=0.0, "Excitation Current Phase Shift I-"=0, "Excitation Current Phase Shift I+"=0, "df frequency quotient"=0.0, "Freqency 0 Deg"=0.0, "Freqency -45 Deg"=0.0, "Freqency +45 Deg"=0.0, "Channel 1 (c1)"=0.0, "Channel 2 (c2)"=0.0, "Coil Temperature"=0.0, "Error State"=0}) -> ()  [unwired: 1 in, 2 out]
            n160 = invoke class="Tbl (strict)" method="Reinit To Default"(reference=w81) -> ()  [unwired: 2 in, 3 out]
            n161 = property class="Enum (strict)"(reference=w68, "Val(Sgnl)"=enum16{"RS-232", "TCP/IP", "Modbus TCP/IP"}."RS-232" ("Value")) -> ()  [unwired: 1 in, 2 out]
            n162 = property class="Clust (strict)"(reference=w67) -> ("Controls[]"=w70:refnum<vi>[])  [unwired: 1 in, 2 out]
            n163 = Index Array(array=w70, index=2) -> (element=w71:refnum<vi>)
            n164 = To More Specific Class(target class=w73, reference=w71) -> (specific class reference=w72:refnum<vi>)  [unwired: 1 in, 1 out]
            n165 = Bundle By Name(cluster=w86, "Stream"="", "Data"=string[][] [] ("initialized array")) -> (w83:T14)
            n166 = call "GetComPortList.vi"() -> ("COM_List"=w74:string[])  [unwired: 10 in, 1 out]
            n167 = property class="CmbBox"(reference=w72, "Strings[]"=w74) -> ()  [unwired: 1 in, 2 out]
          }
          frame "Idle", Default {
            n168 = event shown="[1] \"Connect\": Value Change" {
              selector: w98 -> [_ _ _ _]
              dyn-events: _ -> [_ _ _ _]
              timeout: w96 -> [_ _ _ _]
              tunnel: [_ _ TRUE _] -> w97
              tunnel: [w116 w124 w130 w148] -> w95
              tunnel: w96 -> [w116 w124 w130 w148]
              tunnel: [w112 w121 _ w137] -> w94
              tunnel: [w114 w118 w129 w141] -> w92
              tunnel: w93 -> [w115 w123 w129 w141]
              tunnel: w91 -> [w113 w119 w126 w147]
              tunnel: [w109 w119 w127 w147] -> w90
              event Timeout {
                # "Displaying data if new data important in Modbus Protocal\nTo Avoid Duplicate data"
                # "Reading Data Stream"
                n169 = event-data() -> ()  [unwired: 1 in, 1 out]
                n170 = Unbundle By Name(w115) -> ("ProtocolCls"=w99:refnum<class "Protocol.lvclass">, "StatusLED"=w110:refnum<vi>)
                n171 = call-dynamic "ReadData.vi"("error in (no error)"=w113, "Protocol In"=w99) -> ("error out"=w109:errorcluster, "read buffer"=w105:string, "Protocol Out"=w100:refnum<class "Protocol.lvclass">)  [unwired: 7 in]
                n172 = feedback #1() -> (w106:string)  [unwired: 1 in]
                n173 = feedback-in #1(w105) -> ()
                n174 = Unbundle By Name(w109) -> ("status"=w108:bool)
                n175 = Not Equal?(x=w105, y=w106) -> (x != y?=w104:bool)
                n176 = Not(x=w108) -> (.not. x?=w107:bool)
                n177 = property class="Bool (strict)"(reference=w110, "Value"=w107) -> ()  [unwired: 1 in, 2 out]
                n178 = Bundle By Name(cluster=w115, "ProtocolCls"=w100, "Stream"=w105) -> (w114:T14)
                n179 = Select(t="Display", s=w104, f="Idle") -> (s? t:f=w101:string)
                n180 = Select(t="Error", s=w109, f=w101) -> (s? t:f=w112:string)
              }
              event "Connect": Value Change {
                n181 = event-data() -> ("NewVal"=w117:bool)  [unwired: 1 in]
                n182 = Select(t="OpenConnection", s=w117, f="CloseConnection") -> (s? t:f=w121:string)
                n183 = Bundle By Name(cluster=w123, "ConOpen"=w117) -> (w118:T14)
              }
              event User Event {
                # "Close Communication"
                n184 = event-data() -> ()  [unwired: 1 in, 1 out]
                n185 = Unbundle By Name(w129) -> ("ProtocolCls"=w128:refnum<class "Protocol.lvclass">, "ConOpen"=w125:bool)
                n186 = case shown="True" w125 {
                  tunnel: w128 -> [_ w135]
                  tunnel: [w132 w134] -> w127
                  tunnel: w126 -> [w132 w133]
                  frame False {
                  }
                  frame True {
                    n187 = call-dynamic "CloseConnection.vi"("error in (no error)"=w133, "Protocol In"=w135) -> ("error out"=w134:errorcluster)  [unwired: 8 in, 1 out]
                  }
                }
              }
              event "Protocol": Value Change {
                # "Default Settings After Changing Protocol"
                n188 = event-data() -> ("NewVal"=w142:enum16{"RS-232", "TCP/IP", "Modbus TCP/IP"})  [unwired: 1 in]
                n189 = Unbundle By Name(w141) -> ("ConOpen"=w139:bool, "Com_Set"=w140:refnum<vi>)
                n190 = property class="Clust (strict)"(reference=w140) -> (reference out=w145:refnum<vi>, "Controls[]"=w143:refnum<vi>[])  [unwired: 1 in, 1 out]
                n191 = case shown="\"TCP/IP\"" w142 {
                  tunnel: [bool[] [TRUE, TRUE, FALSE] bool[] [TRUE, TRUE, FALSE] bool[] [FALSE, FALSE, TRUE]] -> w144
                  tunnel: [T5 {"HostName"="localhost", "Port"=10001, "ComPort"=""} ("Com_Set") T5 {"HostName"="localhost", "Port"=502, "ComPort"=""} ("Com_Set") T5 {"HostName"="localhost", "Port"=0, "ComPort"=""} ("Com_Set")] -> w146
                  frame "TCP/IP" {
                  }
                  frame "Modbus TCP/IP" {
                  }
                  frame "RS-232" {
                  }
                }
                n192 = property class="Clust (strict)"(reference=w145, "Value"=w146) -> ()  [unwired: 1 in, 2 out]
                n193 = for {
                  tunnel: w143 -> [w150] mode=indexing
                  tunnel: w144 -> [w149] mode=indexing
                  n194 = property class="Ctl"(reference=w150, "Visible"=w149) -> ()  [unwired: 1 in, 2 out]
                }
                n195 = Select(t="CloseConnection", s=w139, f="Idle") -> (s? t:f=w137:string)
              }
            }
          }
          frame "OpenConnection" {
            # "Open Communication"
            n196 = Unbundle By Name(w160) -> ("Protocol"=w159:refnum<vi>, "Connect"=w158:refnum<vi>, "Com_Set"=w157:refnum<vi>)
            n197 = property class="Enum (strict)"(reference=w159) -> ("Value"=w169:enum16{"RS-232", "TCP/IP", "Modbus TCP/IP"})  [unwired: 1 in, 2 out]
            n198 = property class="Clust (strict)"(reference=w157) -> ("Value"=w170:T1)  [unwired: 1 in, 2 out]
            n199 = call "Protocol_Init.vi"("Protocol"=w169, "error in (no error)"=w164, "Com_Set"=w170) -> ("error out"=w172:errorcluster, "Protocol Out"=w171:refnum<class "Protocol.lvclass">)  [unwired: 7 in]
            n200 = call-dynamic "OpenConnection.vi"("Err In"=w172, "Protocol In"=w171) -> ("Err Out"=w163:errorcluster, "Protocol Out"=w165:refnum<class "Protocol.lvclass">)  [unwired: 8 in]
            n201 = Unbundle By Name(w163) -> ("status"=w162:bool)
            n202 = Bundle By Name(cluster=w160, "ProtocolCls"=w165) -> (w166:T14)
            n203 = Not(x=w162) -> (.not. x?=w161:bool)
            n204 = property class="Bool (strict)"(reference=w158, "Value"=w161) -> ()  [unwired: 1 in, 2 out]
          }
          frame "Display" {
            # "Displaying The Data\nPanel update defer On / Off"
            n205 = Unbundle By Name(w201) -> ("This VI"=w191:refnum<vi>, "LimitRowCount"=w192:u16, "Data"=w193:string[][], "Stream"=w177:string, "Chart1"=w181:refnum<vi>, "Chart2"=w183:refnum<vi>, "Chart3"=w175:refnum<vi>, "LogEnable"=w174:refnum<vi>)
            n206 = property class="Bool (strict)"(reference=w174) -> ("Value"=w173:bool)  [unwired: 1 in, 2 out]
            n207 = call "Convert Received String to Data.vi"("String"=w177) -> ("Cluster"=w176:T2, "Data"=w199:string[])  [unwired: 3 in]
            n208 = case shown="True" w173 {
              tunnel: [w203 w206] -> w187
              tunnel: w186 -> [w203 w205]
              tunnel: w176 -> [_ w204]
              frame False {
              }
              frame True {
                # "Generating Event to log data"
                n209 = call "LogData.vi"("error in"=w205, "Data_Cluster"=w204) -> ("error out"=w206:errorcluster)  [unwired: 9 in]
              }
            }
            n210 = Unbundle By Name(w176) -> ("Resonant Frequency"=w184:dbl, "Damping Frequency"=w185:dbl, "Viscosity"=w179:dbl, "Temperature"=w182:dbl)
            n211 = call "Limit Row Count in Table.vi"("Insert"=w199, "Data_In"=w193, "MaxDataQueue"=w192) -> ("Data_out"=w197:string[][])  [unwired: 8 in]
            n212 = property class="VI"(reference=w191) -> ("Panel"=w196:refnum<vi>)  [unwired: 1 in, 2 out]
            n213 = property class="Pnl"(reference=w196, "DeferPanUpdts"=TRUE ("Defer Panel Updates")) -> (reference out=w190:refnum<vi>)  [unwired: 1 in, 1 out]
            n214 = call "Scale Chart Axis.vi"("V2"=w185, "V1"=w184, "Chart"=w183) -> ("Chart"=w188:cluster{"Viscosity":dbl, "Temperature":dbl})  [unwired: 8 in]
            n215 = call "Scale Chart Axis.vi"("V2"=w182, "V1"=w179, "Chart"=w181) -> ("Chart"=w180:cluster{"Viscosity":dbl, "Temperature":dbl})  [unwired: 8 in]
            n216 = call "Calculate Derivative.vi"("Chart"=w175, "Viscosity"=w179) -> ("Cluster"=w178:cluster{"dx/dt":dbl, "dx/dt":dbl})  [unwired: 9 in]
            n217 = flat-sequence {
              tunnel: w197 -> [w213]
              tunnel: w190 -> [w212]
              tunnel: [w212] -> w189
              tunnel: w188 -> [w211]
              tunnel: w180 -> [w210]
              tunnel: w178 -> [w209]
              tunnel: w177 -> [w208]
              tunnel: w176 -> [w207]
              frame #0 {
                "Table" <- w213
                "Chart2" <- w211
                "Chart1" <- w210
                "Chart3" <- w209
                "ReceivedData" <- w208
                "Data_Cluster" <- w207
              }
            }
            n218 = property class="Pnl"(reference=w189, "DeferPanUpdts"=FALSE ("Defer Panel Updates")) -> ()  [unwired: 1 in, 2 out]
            n219 = Bundle By Name(cluster=w201, "Data"=w197) -> (w198:T14)
          }
          frame "CloseConnection" {
            n220 = Unbundle By Name(w220) -> ("ProtocolCls"=w219:refnum<class "Protocol.lvclass">, "StatusLED"=w217:refnum<vi>, "Connect"=w214:refnum<vi>)
            n221 = call-dynamic "CloseConnection.vi"("Protocol In"=w219) -> ()  [unwired: 9 in, 2 out]
            n222 = property on="Property Node" class="Bool (strict)"(reference=w214, "Value"=FALSE) -> ()  [unwired: 1 in, 2 out]
            n223 = property on="Property Node" class="Bool (strict)"(reference=w217, "Value"=FALSE) -> ()  [unwired: 1 in, 2 out]
          }
          frame "Error" {
            n224 = case shown="Error 63" w226 {
              selector: w226 -> [_ w233 _ _ _ _]
              tunnel: w225 -> [w230 _ _ _ _ w244]
              tunnel: [w230 -1 -1 -1 -1 w244] -> w224
              tunnel: ["Idle" "Idle" "Idle" "Idle" "Idle" "Idle"] -> w223
              frame No Error {
              }
              frame Default {
                n225 = call <vilib>:"Simple Error Handler.vi"("error in (no error)"=w233) -> ()  [unwired: 4 in, 5 out]
              }
              frame Error {
                n226 = One Button Dialog(message="Selected Serial Port not found!") -> ()  [unwired: 1 in, 1 out]
              }
              frame Error {
                n227 = One Button Dialog(message="Select Serial Port First!") -> ()  [unwired: 1 in, 1 out]
              }
              frame Error {
                n228 = One Button Dialog(message="Communication Error!\n1. SME SIM App not running.\n2. Wrong Hostname selection.\n3. Wrong Port number selection.") -> ()  [unwired: 1 in, 1 out]
              }
              frame Error {
              }
            }
          }
        }
        n229 = Select(t="Error", s=w36, f=w34) -> (s? t:f=w33:string)
      }
    }
    frame Error {
      # "Synchronize Caller Events.vi will inform Start Module.vi that the module has launched and will let the code calling Start Module.vi register for broadcasts and would permit the caller receive the broadcast that an error occurred at launch time."
      n230 = call-dynamic "Delacor_lib_QMH_Release Message Queue.vi"("error in"=w515, "Message Queue"=w508) -> ("error out"=w514:errorcluster)  [unwired: 9 in]
      n231 = call "Synchronize Caller Events.vi"("Singleton Module Admin in"=w509) -> ("error out"=w516:errorcluster)  [unwired: 9 in, 1 out]
      n232 = call "Module Name--constant.vi"() -> ("Module Name"=w512:string)  [unwired: 11 in]
      n233 = Format Into String(format string="An error occurred during initialization. %s is no longer running.", w512) -> (resulting string=w510:string)  [unwired: 2 in, 1 out]
      n234 = Merge Errors(w514, w516) -> (w517:errorcluster)
      n235 = call "Error Reported.vi"("Additional Information"=w510, "Error"=w517) -> ()  [unwired: 9 in, 1 out]
    }
  }
  n236 = Merge Errors(w17, w20, w1) -> (w16:errorcluster)
  n237 = call "Close Module.vi"("error in"=w16, "Module Admin in"=w11) -> ("error out"=w18:errorcluster, "External Launch"=w5:bool, "Module Admin out"=w6:refnum<class "Delacor_lib_QMH_Module Admin.lvclass">)  [unwired: 7 in]
  n238 = Unregister For Events(event registration refnum=w10, error in=w18) -> (error out=w15:errorcluster)
  "error out" <- w15
  n239 = case "External Launch?" shown="True" w5 {
    tunnel: w15 -> [_ w518]
    frame False {
    }
    frame True {
      n240 = case shown="Error" w518 {
        frame No Error {
          n241 = invoke on="Invoke Node" class="VI" method="FP.Close"() -> ()  [unwired: 3 in, 3 out]
        }
        frame Error {
          n242 = invoke on="Invoke Node" class="VI" method="FP.Open"("Activate"=TRUE ("Activate?")) -> ()  [unwired: 4 in, 5 out]
        }
      }
    }
  }
  n243 = local write "Module Admin"(w6) -> ()
